vi "Current consumption in seleep mode.vi"(8 "error in":errorcluster) -> (0 "error out":errorcluster, 1 "Pass/Fail":bool, 2 "active":bool, 3 "Imeasured":string, 5 "Isleep":bool)   [LabVIEW 2009]
uses:
  Digit IO PCI 6503/Digit IO control.ctl
  Global/Global 1.vi
  <vilib>/Instr/_visa.llb/VISA Configure Serial Port (Instr).vi
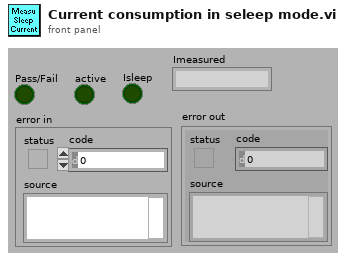
[diagram p1: front panel]
types:
  T1 = typedef "Digit IO control.ctl" = enum16{"Pull X1_4 Low", "Disconnect Pull X1_4 Low", "Down Cylinder", "Disconnect Down Cylinder", "Load X1_1_5", "Disconnect Load X1_1_5", "Measu X1_1_5", "Disconnect Measu X1_1_5", "Measu Z1_1_5", "Disconnect Measu Z1_1_5", "Power X1_1", "Disconnect Power X1_1", "RS232 Power", "Disconnect RS232 Power", "Card Cylinder", "Disconnect Card Cylinder", "Fail LED", "Disconnect Fail LED", "LCA Power", "Disconnect LCA Power", "BeyondCylinderDowndigit", "Disconnect BeyondCylinderDowendigit", "Frequency", "Disconnect Frequency", "Measu Current", "Disconnect Measu Current", "Measu current_1", "Disconnect Measu current_1", "Digit ALL", "Disconnect Digit ALL", "PASS LED", "Disconnect PASS LED", "Load Z1_1_3", "Disconnect Load Z1_1_3", "RS232 Connect", "Disconnect RS232 Connect", "Power Z1_7", "Disconnect Power Z1_7", "Pull Z_1_5  low", "Disconnect Pull Z_1_5  low", "Connect LCA_1", "Disconnect LCA_1", "short LCA", "Disconnect short LCA", "PT100", "Disconnect PT100", "NO connect", "Disconnect NO connect"}
  T2 = cluster{"VHEATFUSENOLOADMIN":string, "VHEATFUSELOADMAX":string, "VOVERRIDEDIODEMIN":string, "TDIFFMAX":string, "MEASFREQMAX":string, "MEASFREQMIN":string, "VOVER":string, "VMIDDLE":string, "VUNDER":string, "VNORESET":string, "VRESET":string, "WAITPING":string, "LRFID":string, "RFIDUID":string, "EXTEESIZE":string, "LCUTYPE":string, "LCUSUBTYPE":string, "TEVN":string, "BOOTVER":string, "APPVER":string, "ISLEEPMAX":string, "TSLEEP":string, "APPWAIT":string, "DBWAIT":string}
  T3 = cluster{"People":string, "product  number":string, "Test time":string, "VHeatFuse_noload":string, "VHeatFuse_load":string, "VoverrideDiode":string, "Test firmware upload via X1":string, "TemperAddress":string, "Troom":string, "TLCU":string, "Adjustment factor":string, "MeasuredFreq":string, "I2C communication":string, "Light-emitting diode on Z2":string, "Battery warning/inhibit":string, "Reset by IC10":string, "External EEPROM":string, "RFID card detection and reading RFID":string, "Production parameters in internal EEPROM":string, "Current consumption in sleep mode":string, "Application and database upload":string, "Test result":string, "Table head[22]":string, "Table head[23]":string}
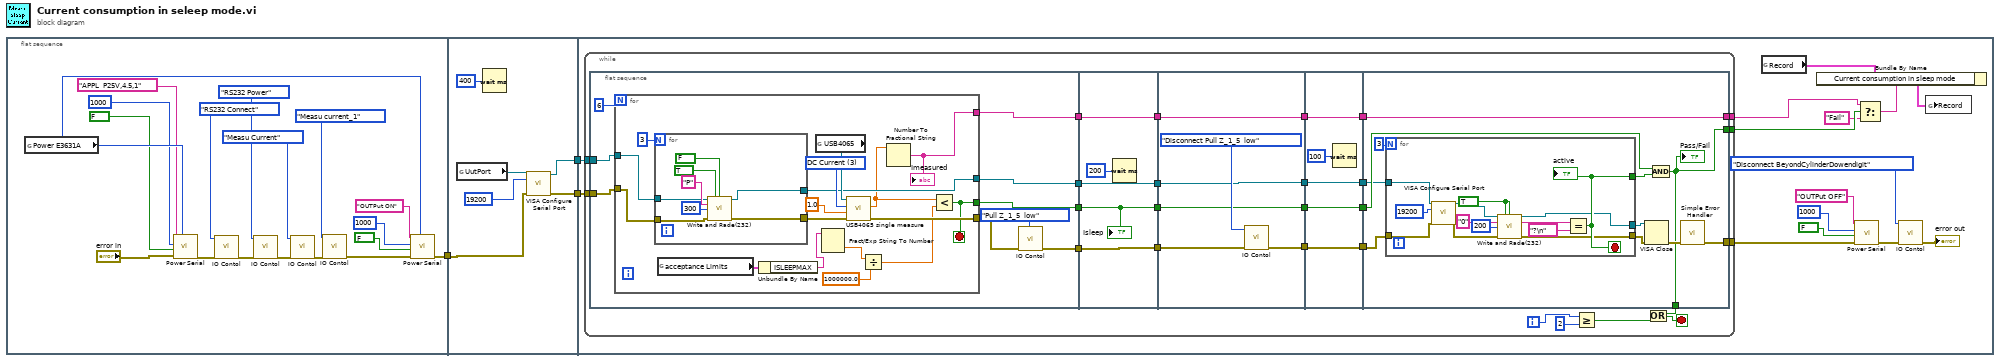
[diagram p0: block diagram]
diagram:
  n1 = flat-sequence {
    tunnel: [w16] -> w3
    tunnel: w3 -> [w23]
    tunnel: [w24] -> w2
    tunnel: [w22] -> w1
    tunnel: w2 -> [w29]
    tunnel: w1 -> [w28]
    frame #0 {
      n2 = global read "Global 1.vi" "Power E3631A"() -> (w18:i32)
      n3 = call "Power Serial.vi"("VISA Resource Address"=w18, "error in (no error)"="error in", "Rd?"=FALSE, "Delay"=1000, "IN"="APPL  P25V,4.5,1" ("In")) -> ("error out"=w10:errorcluster)  [unwired: 6 out]
      n4 = call "IO Contol.vi"("error in"=w10, "IO Operation"=Digit_IO_control."RS232 Connect" ("Enum")) -> ("error out"=w11:errorcluster)  [unwired: 9 out]
      n5 = call "IO Contol.vi"("error in"=w11, "IO Operation"=Digit_IO_control."RS232 Power" ("Enum")) -> ("error out"=w12:errorcluster)  [unwired: 9 out]
      n6 = call "IO Contol.vi"("error in"=w12, "IO Operation"=Digit_IO_control."Measu Current" ("Enum")) -> ("error out"=w9:errorcluster)  [unwired: 9 out]
      n7 = call "IO Contol.vi"("error in"=w9, "IO Operation"=Digit_IO_control."Measu current_1" ("Enum")) -> ("error out"=w17:errorcluster)  [unwired: 9 out]
      n8 = call "Power Serial.vi"("VISA Resource Address"=w18, "error in (no error)"=w17, "Rd?"=FALSE, "Delay"=1000, "IN"="OUTPut ON" ("In")) -> ("error out"=w16:errorcluster)  [unwired: 6 out]
    }
    frame #1 {
      n9 = global read "Global 1.vi" "UutPort"() -> (w26:refnum<visa-resource-name>)
      n10 = Wait (ms)(milliseconds to wait=u32 400) -> ()  [unwired: 1 out]
      n11 = call-poly "VISA Configure Serial Port"("VISA resource name"=w26, "baud rate (9600)"=u32 19200, "error in (no error)"=w23) -> ("VISA resource name out"=w24:refnum<visa-resource-name>, "error out"=w22:errorcluster)  [unwired: 3 in, 8 out]
    }
    frame #2 {
      n12 = while {
        tunnel: [w57] -> w36
        tunnel: [w56] -> w35
        tunnel: [w53] -> w34
        tunnel: w29 -> [w44]
        tunnel: w28 -> [w43]
        i -> [w66]
        stop <- w62 stop-if-true
        n13 = flat-sequence {
          tunnel: [w77] -> w67
          tunnel: [w75] -> w60
          tunnel: [w73] -> w58
          tunnel: [w71] -> w54
          tunnel: w44 -> [w70]
          tunnel: w43 -> [w69]
          tunnel: [w106] -> w68
          tunnel: w67 -> [w106]
          tunnel: [w105] -> w61
          tunnel: w60 -> [w105]
          tunnel: [w104] -> w59
          tunnel: w58 -> [w104]
          tunnel: [w103] -> w55
          tunnel: w54 -> [w103]
          tunnel: w68 -> [w110]
          tunnel: [w113] -> w52
          tunnel: w61 -> [w111]
          tunnel: [w111] -> w50
          tunnel: [w109] -> w48
          tunnel: w59 -> [w109]
          tunnel: [w108] -> w46
          tunnel: w55 -> [w108]
          tunnel: w52 -> [w118]
          tunnel: [w118] -> w51
          tunnel: w50 -> [w117]
          tunnel: [w117] -> w49
          tunnel: w48 -> [w116]
          tunnel: [w116] -> w47
          tunnel: w46 -> [w115]
          tunnel: [w115] -> w45
          tunnel: [w119] -> w64
          tunnel: w51 -> [w129]
          tunnel: w49 -> [w122]
          tunnel: w47 -> [w128]
          tunnel: [w123] -> w57
          tunnel: [w120] -> w56
          tunnel: w45 -> [w120]
          tunnel: [w119] -> w53
          frame #0 {
            n14 = for {
              N: 6 -> [_]
              tunnel: [w91] -> w74
              tunnel: [w89] -> w75
              tunnel: [w88] -> w73
              tunnel: [w86] -> w71
              tunnel: w70 -> [w85]
              tunnel: w69 -> [w84]
              stop <- w88 stop-if-true
              w92 = 3 items=["DC Volts"=1, "AC Volts"=2, "DC Current"=3, "AC Current"=4, "2-Wire Resistance"=5, "4-Wire Resistance"=101, "Frequency"=104, "Period"=105, "AC Volts DC Coupled"=1001, "Diode"=1002, "Waveform Voltage"=1003, "Waveform Current"=1004, "Capacitance"=1005, "Inductance"=1006, "Temperature"=108] ("Configuration:Function")
              n15 = for {
                N: 3 -> [_]
                tunnel: [w102] -> w90
                tunnel: [w101] -> w89
                tunnel: w85 -> [w96]
                tunnel: w84 -> [w95]
                n16 = call "Write and Rade(232).vi"("VISA resource name in"=w96, "write"=TRUE, "read"=FALSE, "string to write"="P", "ms delay"=u32 300 ("millisecond multiple"), "error in"=w95) -> ("VISA resource name out"=w101:refnum<visa-resource-name>, "error out"=w102:errorcluster)  [unwired: 2 in, 6 out]
              }
              n17 = global read "Global 1.vi" "acceptance Limits"() -> (w82:T2)
              n18 = Unbundle By Name(w82) -> ("ISLEEPMAX"=w81:string)
              n19 = global read "Global 1.vi" "USB4065"() -> (w93:refnum<k15>)
              n20 = Fract/Exp String To Number(string=w81) -> (number=w80:dbl)  [unwired: 4 out]
              n21 = call "USB4065 single measure.vi"("error in (no error)"=w90, "Configuration:Range"=1.0, "Configuration:Function"=w92, "Instrument Descriptor"=w93) -> ("error out"=w91:errorcluster, "Measurement"=w87:dbl)  [unwired: 6 out]
              n22 = Divide(x=w80, y=1000000.0) -> (x/y=w78:dbl)
              n23 = Number To Fractional String(number=w87) -> (F-format string=w86:string)  [unwired: 3 out]
              "Imeasured" <- w86
              n24 = Less?(x=w87, y=w78) -> (x < y?=w88:bool)
            }
            n25 = call "IO Contol.vi"("error in"=w74, "IO Operation"=Digit_IO_control."Pull Z_1_5  low" ("Enum")) -> ("error out"=w77:errorcluster)  [unwired: 9 out]
          }
          frame #1 {
            n26 = Wait (ms)(milliseconds to wait=u32 200) -> ()  [unwired: 1 out]
            "Isleep" <- w104
          }
          frame #2 {
            n27 = call "IO Contol.vi"("error in"=w110, "IO Operation"=Digit_IO_control."Disconnect Pull Z_1_5  low" ("Enum")) -> ("error out"=w113:errorcluster)  [unwired: 9 out]
          }
          frame #3 {
            n28 = Wait (ms)(milliseconds to wait=u32 100) -> ()  [unwired: 1 out]
          }
          frame #4 {
            n29 = for {
              N: 3 -> [_]
              tunnel: w129 -> [w131]
              tunnel: [w138] -> w127
              tunnel: [w137] -> w125
              tunnel: w122 -> [w135]
              tunnel: [w136] -> w121
              stop <- w138 stop-if-true
              w139 = TRUE ("write")
              n30 = call-poly "VISA Configure Serial Port"("VISA resource name"=w135, "baud rate (9600)"=u32 19200, "error in (no error)"=w131) -> ("VISA resource name out"=w134:refnum<visa-resource-name>, "error out"=w132:errorcluster)  [unwired: 3 in, 8 out]
              n31 = call "Write and Rade(232).vi"("VISA resource name in"=w134, "write"=w139, "read"=w139, "string to write"="0", "ms delay"=u32 200, "error in"=w132) -> ("VISA resource name out"=w136:refnum<visa-resource-name>, "read string"=w140:string, "error out"=w137:errorcluster)  [unwired: 2 in, 5 out]
              n32 = Equal?(x=w140, y="?\n") -> (x = y?=w138:bool)
              "active" <- w138
            }
            n33 = VISA Close(VISA resource name=w121, error in (no error)=w125) -> (error out=w124:errorcluster)
            n34 = And(x=w128, y=w127) -> (x .and. y?=w119:bool)
            "Pass/Fail" <- w119
            n35 = call <vilib>:"Simple Error Handler.vi"("error in (no error)"=w124) -> ("error out"=w123:errorcluster)  [unwired: 1 in, 7 out]
          }
        }
        n36 = Greater Or Equal?(x=w66, y=2) -> (x >= y?=w63:bool)
        n37 = Or(x=w64, y=w63) -> (x .or. y?=w62:bool)
      }
      n38 = global read "Global 1.vi" "Record"() -> (w32:T3)
      n39 = call "Power Serial.vi"("error in (no error)"=w36, "Rd?"=FALSE, "Delay"=1000, "IN"="OUTPut OFF" ("In")) -> ("error out"=w39:errorcluster)  [unwired: 1 in, 6 out]
      n40 = Select(t=w35, s=w34, f="Fail") -> (s? t:f=w31:string)
      n41 = Bundle By Name(cluster=w32, "Current consumption in sleep mode"=w31) -> (w30:T3)
      n42 = call "IO Contol.vi"("error in"=w39, "IO Operation"=Digit_IO_control."Disconnect BeyondCylinderDowendigit" ("Enum")) -> ("error out"=→"error out":errorcluster)  [unwired: 9 out]
      n43 = global write "Global 1.vi" "Record"(w30) -> ()
    }
  }
